vi "TSP-搜索树形列表（表格）.vi"(8 "error in (no error)":errorcluster caption="错误输入（无错误）") -> (0 "错误输出":errorcluster, 2 "项缩进层次":i32[](array[numeric]), 3 "项名称":string[](array[string]), 4 "All Files in Dir":path[](array[path]) caption="目录中的所有文件", 5 "文件夹名":string[](array[string]))   [LabVIEW 2017]
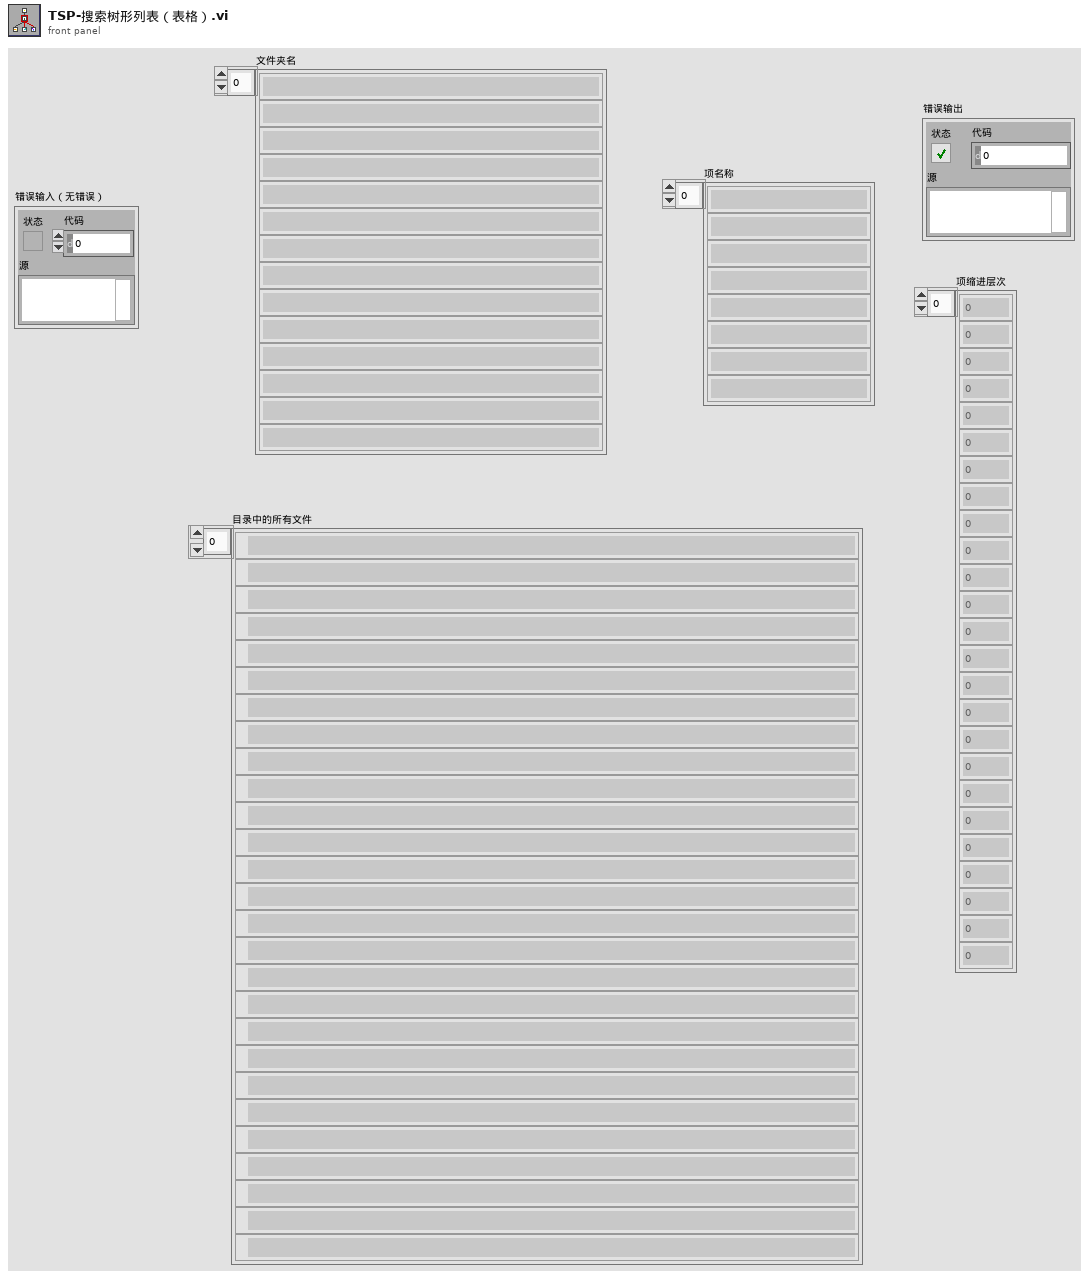
[diagram p1: front panel]
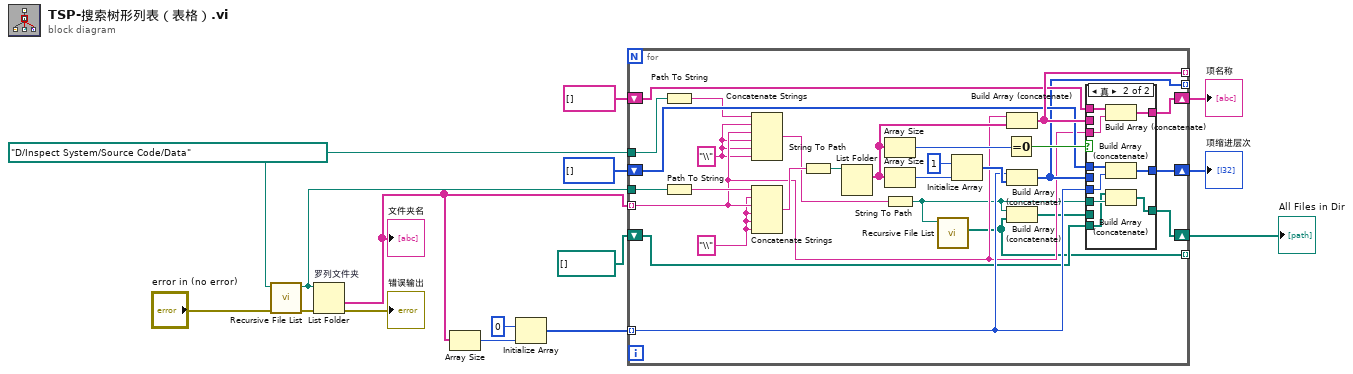
[diagram p0: block diagram]
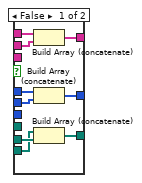
[diagram p2: hidden frame]
diagram:
  w2 = path "D:/Inspect System/Source Code/Data" ("Folder Path")
  n1 = call <vilib>:"Recursive File List.vi"("error in (no error)"="error in (no error)", "Folder Path"=w2) -> ("error out"=w15:errorcluster, "dup Folder Path"=w14:path)  [unwired: 5 in, 3 out]
  n2 = List Folder "罗列文件夹"(path=w14, error in=w15) -> (folder names=w13:string[], error out=→"错误输出":errorcluster)  [unwired: 2 in, 2 out]
  "文件夹名" <- w13
  n3 = Array Size(array=w13) -> (size(s)=w10:i32)
  n4 = Initialize Array(0 ("维数大小"), w10) -> (w12:i32[])
  n5 = for {
    tunnel: w13 -> [w22] mode=indexing
    tunnel: w14 -> [w43]
    tunnel: [w32] -> _ mode=indexing
    tunnel: w12 -> [w27] mode=indexing
    tunnel: [w28] -> _ mode=indexing
    shift-right: [w33] -> w8
    shift-left: string[] [] -> [w31]
    shift-right: [w29] -> w6
    shift-left: i32[] [] -> [w30]
    shift-right: [w25] -> w1
    shift-left: path[] [] -> [w26]
    tunnel: w2 -> [w24]
    tunnel: [w20] -> _ mode=indexing
    w16 = "\\" ("字符串")
    w17 = "\\" ("字符串")
    n6 = Path To String(path=w24) -> (string=w23:string)
    n7 = Path To String(path=w43) -> (string=w42:string)
    n8 = Concatenate Strings(w23, w16, w22, w16, w16, w16) -> (w21:string)
    n9 = Concatenate Strings(w42, w17, w22, w17, w17, w17) -> (w41:string)
    n10 = String To Path(string=w41) -> (path=w40:path)
    n11 = List Folder(path=w40) -> (filenames=w35:string[])  [unwired: 3 in, 3 out]
    n12 = Array Size(array=w35) -> (size(s)=w36:i32)
    n13 = Array Size(array=w35) -> (size(s)=w37:i32)
    n14 = String To Path(string=w21) -> (path=w19:path)
    n15 = call <vilib>:"Recursive File List.vi"("Folder Path"=w19) -> ("All Files in Dir"=w20:path[])  [unwired: 6 in, 4 out]
    n16 = Initialize Array(1 ("维数大小"), w37) -> (w39:i32[])
    n17 = Equal To 0?(x=w36) -> (x = 0?=w34:bool)
    n18 = Build Array (concatenate)(w22, w35) -> (w32:string[])
    n19 = Build Array (concatenate)(w27, w39) -> (w28:i32[])
    n20 = Build Array (concatenate)(w19, w20) -> (w18:path[])
    n21 = case shown="真" w34 {
      tunnel: w31 -> [w52 w60]
      tunnel: [w50 w59] -> w33
      tunnel: w32 -> [w51 _]
      tunnel: w30 -> [w48 w57]
      tunnel: [w47 w56] -> w29
      tunnel: w28 -> [w49 _]
      tunnel: w22 -> [_ w61]
      tunnel: w27 -> [_ w58]
      tunnel: w26 -> [w45 w54]
      tunnel: [w44 w53] -> w25
      tunnel: w19 -> [_ w55]
      tunnel: w18 -> [w46 _]
      frame False {
        n22 = Build Array (concatenate)(w52, w51) -> (w50:string[])
        n23 = Build Array (concatenate)(w48, w49) -> (w47:i32[])
        n24 = Build Array (concatenate)(w45, w46) -> (w44:path[])
      }
      frame True {
        n25 = Build Array (concatenate)(w60, w61) -> (w59:string[])
        n26 = Build Array (concatenate)(w57, w58) -> (w56:i32[])
        n27 = Build Array (concatenate)(w54, w55) -> (w53:path[])
      }
    }
  }
  "项名称" <- w8
  "项缩进层次" <- w6
  "All Files in Dir" <- w1
